vi "M03 Hybrid Car.vi"(11 "EV3 in":T1) -> (3 "EV3 out":T1)   [LabVIEW 2016]
uses:
  <vilib>/NXT/Subs/LVHSConnector.ctl
  <vilib>/NXT/LegoClasses/BrickReference/BrickReference.lvclass
  <vilib>/NXT/Block Support/NXT_OutputPort.ctl
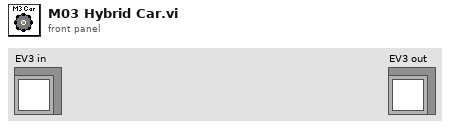
[diagram p1: front panel]
types:
  T1 = typedef "LVHSConnector.ctl" = refnum<class "BrickReference.lvclass">
  T2 = typedef "NXT_OutputPort.ctl" = u8
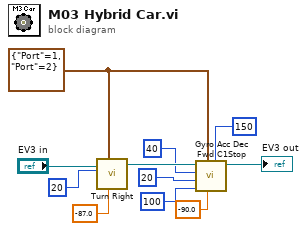
[diagram p0: block diagram]
diagram:
  w3 = cluster{"Port":T2, "Port":T2} {"Port"=1, "Port"=2} ("Motor")
  n1 = call "Turn Right.vi"("Turning angle"=sgl -87.0, "Motor"=w3, "Motor B (right)"=i8 20, "EV3 in"="EV3 in") -> ("EV3 out"=w9:T1)  [unwired: 7 in]
  n2 = call "Gyro Acc Dec Fwd C1Stop.vi"("Threshold to C1"=150, "Ini. Degrees"=sgl -90.0, "Motor"=w3, "Threshold to De-acc"=100, "De-acc"=20, "Acc"=40, "EV3 in"=w9) -> ("EV3 out"=→"EV3 out":T1)  [unwired: 4 in]
